vi "Array Point to RowCol.vi"(6 "Element Gap?":bool, 7 "Border Width":i32(ring)=3 items=["Classic"=3, "Modern"=4], 8 "error in (no error)":errorcluster, 9 "Mouse Coords":cluster{"Horizontal":i32, "Vertical":i32}, 11 "Array Ref":refnum<vi>) -> (0 "error out":errorcluster, 1 "Clicked Index":i32[](array[numeric]), 2 "Within Bounds?":bool, 3 "dup Ref":refnum<vi>)   [LabVIEW 2023]
doc: "Converts a pixel coordinate to an index into the array. Returns an array of indices with a length equal to the number of dimensions in the array. This method also returns whether the point is inside the bounds of the content rectangle.\n\nWritten by J. David Saunders"
panel:
  # "Written by J. David Saunders"
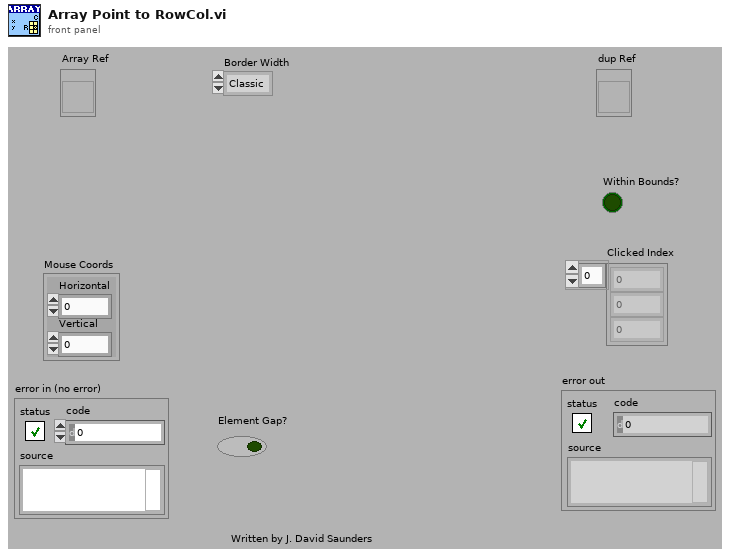
[diagram p1: front panel]
types:
  T1 = typedef "LVBoundsTypeDef.ctl" = cluster{"Width":u32, "Height":u32}
  T2 = cluster{"Number of Columns":u32, "Number of Rows":u32}
  T3 = cluster{"Number of Columns":i32, "Number of Rows":i32}
  T4 = typedef "LVPositionTypeDef.ctl" = cluster{"Left":i32, "Top":i32}
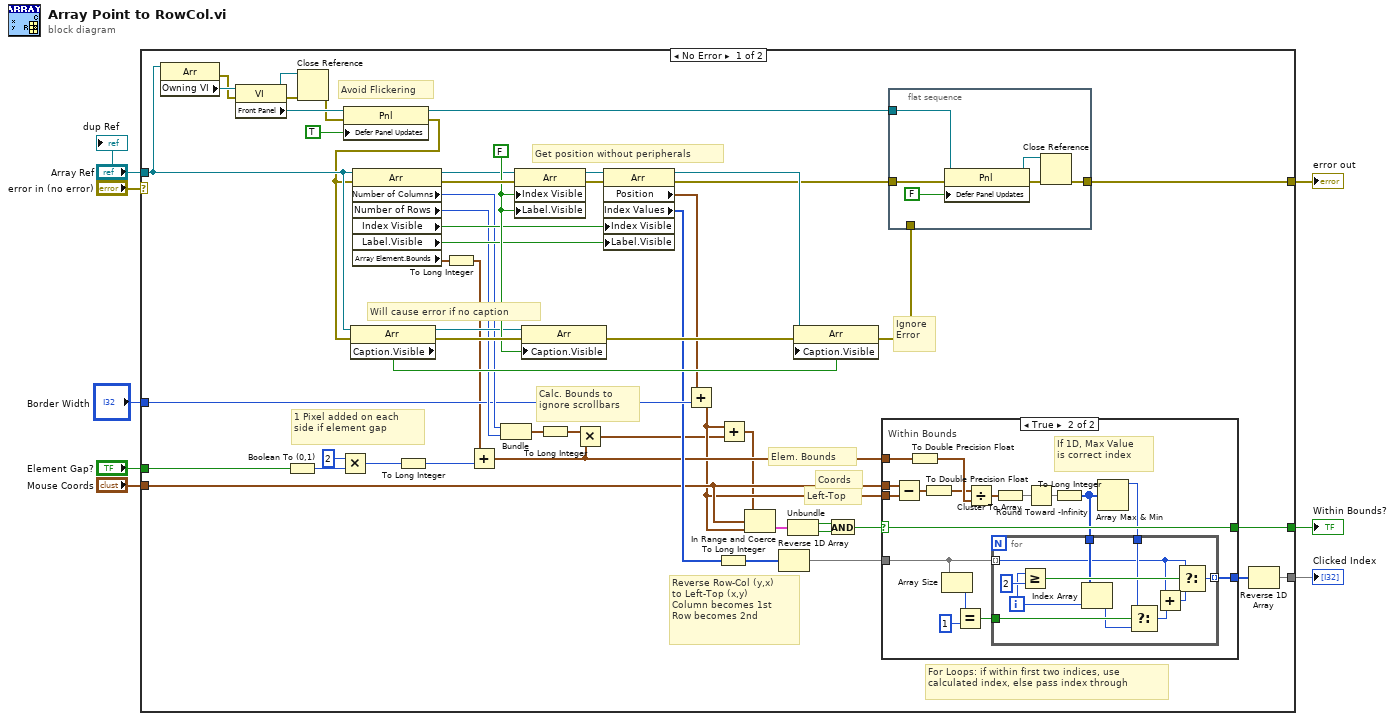
[diagram p0: block diagram]
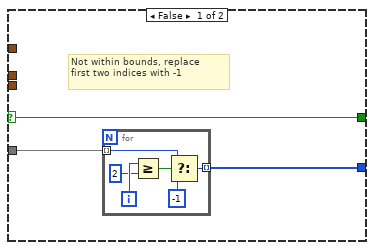
[diagram p2: hidden frame]
diagram:
  n1 = case shown="No Error" "error in (no error)" {
    selector: "error in (no error)" -> [_ w105]
    tunnel: "Element Gap?" -> [w61 _]
    tunnel: "Array Ref" -> [w22 _]
    tunnel: "Mouse Coords" -> [w31 _]
    tunnel: "Border Width" -> [w40 _]
    tunnel: [w35 _] -> w3
    tunnel: [w15 w105] -> w2
    tunnel: [w28 _] -> w1
    frame No Error {
      w56 = FALSE
      # "Avoid Flickering"
      # "Calc. Bounds to\nignore scrollbars"
      # "For Loops: if within first two indices, use\ncalculated index, else pass index through"
      # "Reverse Row-Col (y,x)\nto Left-Top (x,y)\nColumn becomes 1st\nRow becomes 2nd"
      # "Left-Top"
      # "Coords"
      # "Elem. Bounds"
      # "Ignore\nError"
      # "Get position without peripherals"
      # "1 Pixel added on each\nside if element gap"
      # "Will cause error if no caption"
      n2 = property class="Arr"(reference=w22) -> (error out=w20:errorcluster, "Owning VI"=w23:refnum<vi>)  [unwired: 1 in, 1 out]
      n3 = property class="VI"(reference=w23, error in=w20) -> (reference out=w11:refnum<vi>, error out=w10:errorcluster, "Front Panel"=w24:refnum<vi>)
      n4 = Boolean To (0,1)(Boolean=w61) -> (0, 1=w60:i16)
      n5 = Close Reference(reference=w11, error in (no error)=w10) -> (error out=w9:errorcluster)
      n6 = Multiply(x=i16 2 ("y"), y=w60) -> (x*y=w45:i16)
      n7 = property class="Pnl"(reference=w24, error in=w9, "Defer Panel Updates"=TRUE) -> (reference out=w18:refnum<vi>, error out=w19:errorcluster)
      n8 = property class="Arr"(reference=w22, error in=w19) -> (reference out=w50:refnum<vi>, error out=w58:errorcluster, "Caption.Visible"=w47:bool)
      n9 = property class="Arr"(reference=w22, error in=w19) -> (reference out=w53:refnum<vi>, error out=w57:errorcluster, "Number of Columns"=w44:u32, "Number of Rows"=w43:u32, "Index Visible"=w55:bool, "Label.Visible"=w54:bool, "Array Element.Bounds"=w46:T1)
      n10 = To Long Integer(number=w45) -> (32bit integer=w14:i32)
      n11 = To Long Integer(number=w46) -> (32bit integer=w13:cluster{"Width":i32, "Height":i32})
      n12 = Add(x=w13, y=w14) -> (x+y=w30:cluster{"Width":i32, "Height":i32})
      n13 = Bundle("Number of Columns"=w44, "Number of Rows"=w43) -> (w42:T2)  [unwired: 1 in]
      n14 = property class="Arr"(reference=w53, error in=w57, "Index Visible"=w56, "Label.Visible"=w56) -> (reference out=w52:refnum<vi>, error out=w51:errorcluster)
      n15 = property class="Arr"(reference=w50, error in=w58, "Caption.Visible"=w56) -> (error out=w48:errorcluster)  [unwired: 1 out]
      n16 = To Long Integer(number=w42) -> (32bit integer=w12:T3)
      n17 = Multiply(x=w12, y=w30) -> (x*y=w26:cluster{i32, i32})
      n18 = property class="Arr"(reference=w52, error in=w51, "Index Visible"=w55, "Label.Visible"=w54) -> (reference out=w49:refnum<vi>, error out=w17:errorcluster, "Position"=w41:T4, "Index Values"=w34:u32[])
      n19 = Add(x=w41, y=w40) -> (x+y=w27:T4)
      n20 = To Long Integer(number=w34) -> (32bit integer=w32:i32[])
      n21 = Add(x=w27, y=w26) -> (x+y=w25:T4)
      n22 = In Range and Coerce(upper limit=w25, x=w31, lower limit=w27) -> (In Range?=w39:cluster{"Left":bool, "Top":bool})  [unwired: 1 out]
      n23 = Reverse 1D Array(array=w32) -> (reversed array=w33:i32[])
      n24 = Unbundle(w39) -> ("Left"=w38:bool, "Top"=w37:bool)
      n25 = property class="Arr"(reference=w49, error in=w48, "Caption.Visible"=w47) -> (error out=w16:errorcluster)  [unwired: 1 out]
      n26 = And(x=w38, y=w37) -> (x .and. y?=w36:bool)
      n27 = case "Within Bounds" shown="True" w36 {
        selector: w36 -> [w70 w93]
        tunnel: [w70 w93] -> w35
        tunnel: w33 -> [w69 w84]
        tunnel: w31 -> [_ w92]
        tunnel: w30 -> [_ w89]
        tunnel: w27 -> [_ w91]
        tunnel: [w68 w87] -> w29
        frame False {
          # "Not within bounds, replace\nfirst two indices with -1"
          n28 = for {
            tunnel: w69 -> [w73] mode=indexing
            tunnel: [w71] -> w68 mode=indexing
            i -> [w76]
            n29 = Greater Or Equal?(x=w76, y=2) -> (x >= y?=w74:bool)
            n30 = Select(t=w73, s=w74, f=-1) -> (s? t:f=w71:i32)
          }
        }
        frame True {
          # "If 1D, Max Value\nis correct index"
          n31 = Subtract(x=w92, y=w91) -> (x-y=w90:T4)
          n32 = To Double Precision Float(number=w89) -> (double precision float=w78:cluster{"Width":dbl, "Height":dbl})
          n33 = To Double Precision Float(number=w90) -> (double precision float=w77:cluster{"Left":dbl, "Top":dbl})
          n34 = Array Size(array=w84) -> (size(s)=w83:i32)
          n35 = Equal?(x=w83, y=1) -> (x = y?=w81:bool)
          n36 = Divide(x=w77, y=w78) -> (x/y=w88:cluster{dbl, dbl})
          n37 = Cluster To Array(cluster=w88) -> (array=w80:dbl[])
          n38 = Round Toward -Infinity(1:w80) -> (0:w79:dbl[])
          n39 = To Long Integer(number=w79) -> (32bit integer=w86:i32[])
          n40 = Array Max & Min(array=w86) -> (max value=w85:i32)  [unwired: 3 out]
          n41 = for {
            tunnel: w84 -> [w95] mode=indexing
            tunnel: w86 -> [w101]
            tunnel: [w102] -> w87 mode=indexing
            tunnel: w85 -> [w98]
            tunnel: w81 -> [w99]
            i -> [w100]
            n42 = Greater Or Equal?(x=w100, y=2) -> (x >= y?=w103:bool)
            n43 = Index Array(array=w101, index=w100) -> (element=w97:i32)
            n44 = Select(t=w98, s=w99, f=w97) -> (s? t:f=w96:i32)
            n45 = Add(x=w95, y=w96) -> (x+y=w94:i32)
            n46 = Select(t=w95, s=w103, f=w94) -> (s? t:f=w102:i32)
          }
        }
      }
      n47 = flat-sequence {
        tunnel: w18 -> [w65]
        tunnel: w17 -> [w66]
        tunnel: w16 -> [_]
        tunnel: [w63] -> w15
        frame #0 {
          n48 = property class="Pnl"(reference=w65, error in=w66, "Defer Panel Updates"=FALSE) -> (reference out=w62:refnum<vi>, error out=w64:errorcluster)
          n49 = Close Reference(reference=w62, error in (no error)=w64) -> (error out=w63:errorcluster)
        }
      }
      n50 = Reverse 1D Array(array=w29) -> (reversed array=w28:i32[])
    }
    frame Error {
    }
  }
  "Clicked Index" <- w1
  "Within Bounds?" <- w3
  "error out" <- w2
  "dup Ref" <- "Array Ref"
